vi "Count by Status.vi"(10 "Status":T1, 11 "Test Suite Result in":refnum<class "Test Suite Result.lvclass">) -> (2 "Count":i32, 3 "Test Suite Result out":refnum<class "Test Suite Result.lvclass">)   [LabVIEW 2020, in "Test Suite Result.lvclass"]
uses:
  Test Suite Result.lvclass
  Assertion Result/Public/TypeDefs/Status.ctl
  Test Suite Result.lvclass/Test Suite Result.ctl
  Test Case Result/Test Case Result.lvclass/Test Case Result.ctl
  Method Result/Method Result.lvclass/Method Result.ctl
  Test Case Result/Private/SubVIs/Merge Status.vi
  Test Case Result/Test Case Result.lvclass
  Assertion Result/Assertion Result.lvclass
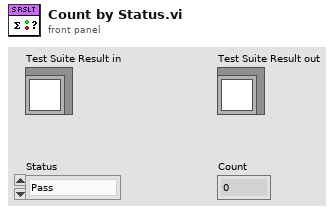
[diagram p1: front panel]
types:
  T1 = typedef "Assertion Result.lvclass/Status.ctl" = enum16{"Pass", "Fail", "Error", "Skipped", "Setup Error", "Broken", "Teardown Error"}
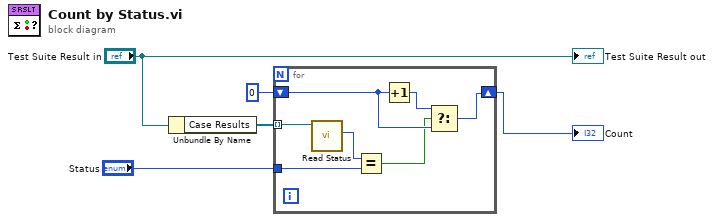
[diagram p0: block diagram]
diagram:
  n1 = Unbundle By Name("Test Suite Result in") -> ("Case Results"=w1:refnum<class "Test Case Result.lvclass">[])
  n2 = for {
    tunnel: w1 -> [w12] mode=indexing
    tunnel: "Status" -> [w10]
    shift-right: [w7] -> w5
    shift-left: 0 -> [w8]
    n3 = call "Read Status.vi"("Test Case Result In"=w12) -> ("Status"=w11:T1)  [unwired: 8 in, 2 out]
    n4 = Equal?(x=w11, y=w10) -> (x = y?=w6:bool)
    n5 = Increment(x=w8) -> (x+1=w9:i32)
    n6 = Select(t=w9, s=w6, f=w8) -> (s? t:f=w7:i32)
  }
  "Count" <- w5
  "Test Suite Result out" <- "Test Suite Result in"
